vi "TEST_TankControl18V7.vi"() -> ()   [LabVIEW 2024]
doc: "This example performs writes and reads on a serial port, as directed by the user. You can press the Write and Read buttons, and change the Read Count, while the example is running.\n\nThe parameters set for the serial port must match the parameters of the connected instrument or device. In this example, the Read Count parameter specifies the number of bytes that the serial port reads. If there were more bytes at the port than the specified number, those bytes would not be read. If there were less bytes at the port than the specified number, you would receive a timeout error.\n\nThis example expands upon the flow control options for XON and XOFF, allowing the user to choose those control characters. Also, the user can enable or disable a termination character. Some devices require a termination character in order to identify the end of command strings. Some devices send a termination character to signify the end of data to be read. This example shows how you can end the Read operation once a termination character is detected in the buffer and/or append a termination character at the end of the Write data."
uses:
  LabVIEW_InstrDriver_forLK-G3000_ver1_0_1_0/32bit/Keyence LK-G3000/Public/clusters/LKIF_FLOATVALUE.ctl
  LabVIEW_InstrDriver_forLK-G3000_ver1_0_1_0/32bit/Keyence LK-G3000/Public/enums/LKIF_FLOATRESULT.ctl
  <vilib>/Instr/_visa.llb/VISA Configure Serial Port (Instr).vi
  LabVIEW_InstrDriver_forLK-G3000_ver1_0_1_0/32bit/Keyence LK-G3000/Keyence LK-G3000.lvlib
panel:
  out "ComCmd":string
  in  "Enable Laser":bool
  in  "Enable \nDout Msg":bool
  in  "Timer ON":bool
  in  "Set Time (sec)":dbl=60.0 format="%#_13g"
  out "Time out":dbl
  out "Value 2":sgl=-inf
  out "Value":sgl=4.5686
  out "Pump State Out":enum16{"INIT", "IDLE", "STOP", "FILL", "DRAIN"}(ring)=enum."STOP"
  out "Cmd Out":u32=56 format="%x"
  in  "Pump Speed":enum16{"FAST", "SLOW", "CREEP", "STOP"}(ring)=enum."SLOW"
  out "CalcData2":T1={"LKIF_FLOATRESULT"=2, "Value"=-inf} {"LKIF_FLOATRESULT" items=["VALID", "RANGEOVER_P", "RANGEOVER_N", "WAITING"]}
  out "CalcData1":T1={"LKIF_FLOATRESULT"=0, "Value"=4.5686} {"LKIF_FLOATRESULT" items=["VALID", "RANGEOVER_P", "RANGEOVER_N", "WAITING"]}
  in  "DRAIN":bool
  in  "FILL":bool
  in  "Stop Button":bool
  # "CMD TABLE"
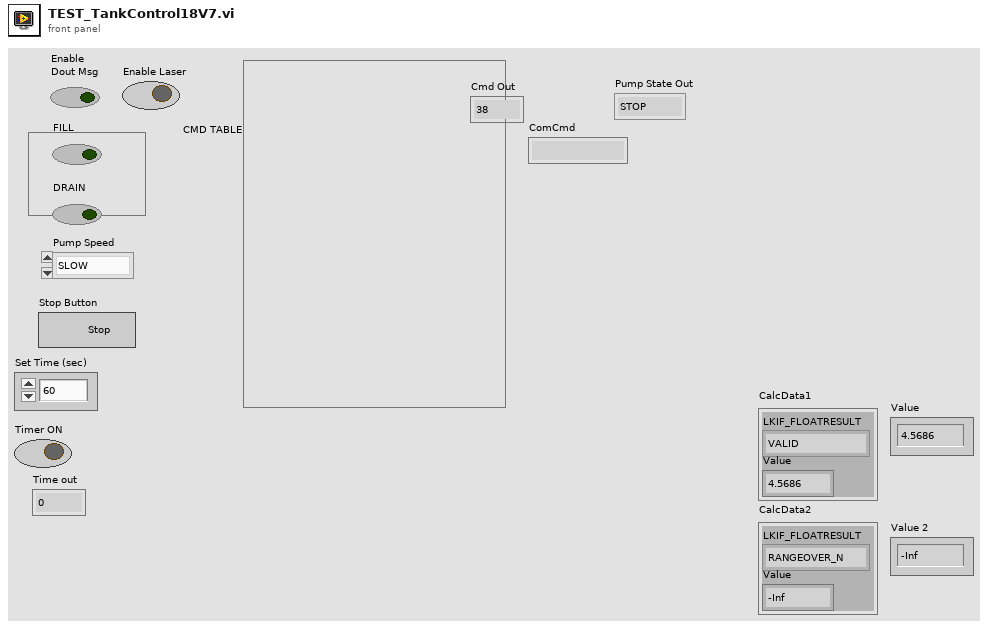
[diagram p1: front panel]
types:
  T1 = typedef "Keyence LK-G3000.lvlib/LKIF_FLOATVALUE.ctl" = cluster{"LKIF_FLOATRESULT":T2, "Value":sgl}
  T2 = typedef "Keyence LK-G3000.lvlib/LKIF_FLOATRESULT.ctl" = i32
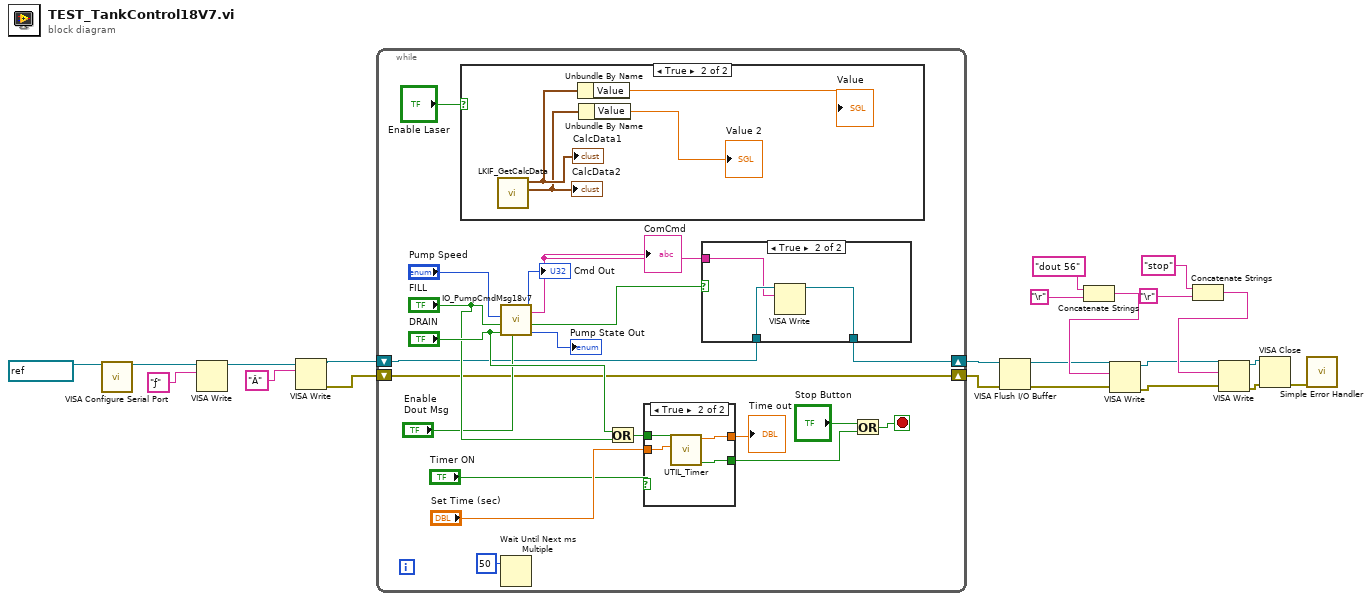
[diagram p0: block diagram]
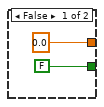
[diagram p3: hidden frame]
diagram:
  n1 = call-poly "VISA Configure Serial Port"("VISA resource name"=refnum<visa-resource-name> "COM4") -> ("VISA resource name out"=w4:refnum<visa-resource-name>)  [unwired: 13 in, 1 out]
  n2 = VISA Write(VISA resource name=w4, write buffer="ƒ") -> (VISA resource name out=w3:refnum<visa-resource-name>)  [unwired: 1 in, 2 out]
  n3 = VISA Write(VISA resource name=w3, write buffer="Â") -> (VISA resource name out=w2:refnum<visa-resource-name>, error out=w1:errorcluster)  [unwired: 1 in, 1 out]
  n4 = while {
    shift-right: [w25] -> w18
    shift-left: w2 -> [w26]
    shift-right: [w27] -> w17
    shift-left: w1 -> [w27]
    stop <- w35 stop-if-true
    n5 = case shown="True" "Enable Laser" {
      frame False {
      }
      frame True {
        n6 = call "LKIF_GetCalcData.vi"() -> ("CalcData2"=w55:T1, "CalcData1"=w56:T1)  [unwired: 9 in, 1 out]
        "CalcData1" <- w56
        "CalcData2" <- w55
        n7 = Unbundle By Name(w56) -> ("Value"=→"Value":sgl)
        n8 = Unbundle By Name(w55) -> ("Value"=→"Value 2":sgl)
      }
    }
    n9 = call "IO_PumpCmdMsg18v7.vi"("Enable"="Enable \nDout Msg", "Drain Signal"="DRAIN", "FIll Signal"="FILL", "Pump Speed"="Pump Speed") -> ("Pump State Out"=→"Pump State Out":enum16{"INIT", "IDLE", "STOP", "FILL", "DRAIN"}, "Msg Active"=w24:bool, "Cmd Out"=→"Cmd Out":u32, "ComCmd"=w23:string)  [unwired: 4 in]
    "ComCmd" <- w23
    n10 = Wait Until Next ms Multiple(millisecond multiple=50) -> ()  [unwired: 1 out]
    n11 = Or(x="DRAIN", y="FILL") -> (x .or. y?=w38:bool)
    n12 = case shown="True" "Timer ON" {
      tunnel: w38 -> [_ w52]
      tunnel: [FALSE ("Timed Out") w51] -> w33
      tunnel: [0.0 ("Numeric") w50] -> w32
      tunnel: "Set Time (sec)" -> [_ w49]
      frame False {
      }
      frame True {
        n13 = call "UTIL_Timer.vi"("Time (sec)"=w49, "Start"=w52) -> ("Timed Out"=w51:bool, "Numeric"=w50:dbl)  [unwired: 4 in, 4 out]
      }
    }
    "Time out" <- w32
    n14 = case shown="True" w24 {
      tunnel: w23 -> [_ w44]
      tunnel: w26 -> [w43 w46]
      tunnel: [w43 w45] -> w25
      frame False {
      }
      frame True {
        n15 = VISA Write(VISA resource name=w46, write buffer=w44) -> (VISA resource name out=w45:refnum<visa-resource-name>)  [unwired: 1 in, 2 out]
      }
    }
    n16 = Or(x="Stop Button", y=w33) -> (x .or. y?=w35:bool)
  }
  n17 = VISA Flush I/O Buffer(VISA resource name=w18, error in (no error)=w17) -> (VISA resource name out=w16:refnum<visa-resource-name>, error out=w15:errorcluster)  [unwired: 1 in]
  n18 = Concatenate Strings("dout 56", "\r") -> (w19:string)
  n19 = VISA Write(VISA resource name=w16, write buffer=w19, error in (no error)=w15) -> (VISA resource name out=w11:refnum<visa-resource-name>, error out=w10:errorcluster)  [unwired: 1 out]
  n20 = Concatenate Strings("stop", "\r") -> (w12:string)
  n21 = VISA Write(VISA resource name=w11, write buffer=w12, error in (no error)=w10) -> (VISA resource name out=w9:refnum<visa-resource-name>, error out=w8:errorcluster)  [unwired: 1 out]
  n22 = VISA Close(VISA resource name=w9, error in (no error)=w8) -> (error out=w22:errorcluster)
  n23 = call <vilib>:"Simple Error Handler.vi"("error in (no error)"=w22) -> ()  [unwired: 1 in, 8 out]
